vi "Read files V CH1(Recorder).vi"(10 "Path":path, 11 "Number":dbl) -> (3 "Voltage":dbl format="%_5g")   [LabVIEW 2020, in "GPP.lvlib"]
uses:
  GPP.lvlib
panel:
  out "String":string
  out "String 2":string
  out "String 3":string
  out "Array":u8[](array[numeric])
  out "Numeric":u16
  out "V1 2":string
  out "V1":string
  out "LAST1":string
  out "SET":string
  out "ALL":string
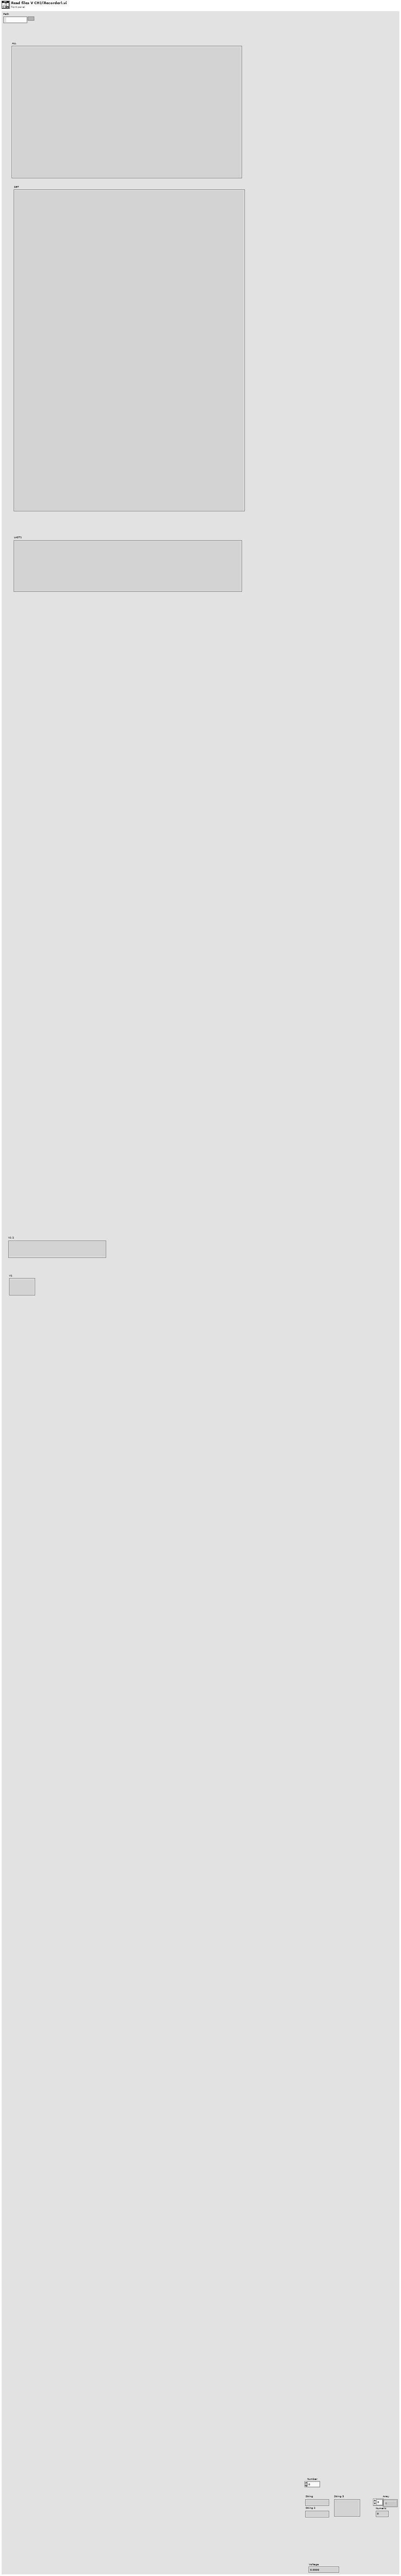
[diagram p1: front panel]
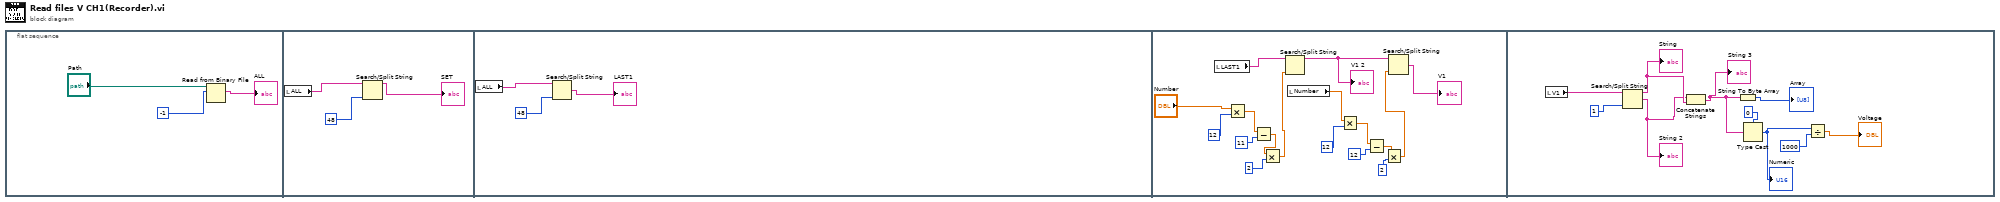
[diagram p0: block diagram]
diagram:
  n1 = flat-sequence {
    frame #0 {
      n2 = Read from Binary File(10:-1, 11:"Path") -> (2:→"ALL":string)  [unwired: 4 in, 3 out]
    }
    frame #1 {
      n3 = local read "ALL"() -> (w4:string)
      n4 = Search/Split String(string=w4, offset (0)=48) -> (substring before match=→"SET":string)  [unwired: 1 in, 2 out]
    }
    frame #2 {
      n5 = local read "ALL"() -> (w7:string)
      n6 = Search/Split String(string=w7, offset (0)=48) -> (match + rest of string=→"LAST1":string)  [unwired: 1 in, 2 out]
    }
    frame #3 {
      n7 = local read "LAST1"() -> (w23:string)
      n8 = Multiply(x="Number", y=12) -> (x*y=w22:dbl)
      n9 = Subtract(x=w22, y=11) -> (x-y=w15:dbl)
      n10 = Multiply(x=w15, y=2) -> (x*y=w13:dbl)
      n11 = Search/Split String(string=w23, offset (0)=w13) -> (substring before match=w16:string)  [unwired: 1 in, 2 out]
      "V1 2" <- w16
      n12 = local read "Number"() -> (w17:dbl)
      n13 = Multiply(x=w17, y=12) -> (x*y=w19:dbl)
      n14 = Subtract(x=w19, y=12) -> (x-y=w12:dbl)
      n15 = Multiply(x=w12, y=2) -> (x*y=w10:dbl)
      n16 = Search/Split String(string=w16, offset (0)=w10) -> (match + rest of string=→"V1":string)  [unwired: 1 in, 2 out]
    }
    frame #4 {
      n17 = local read "V1"() -> (w36:string)
      n18 = Search/Split String(string=w36, offset (0)=1) -> (substring before match=w34:string, match + rest of string=w33:string)  [unwired: 1 in, 1 out]
      "String" <- w34
      "String 2" <- w33
      n19 = Concatenate Strings(w33, w34) -> (w31:string)
      "String 3" <- w31
      n20 = String To Byte Array(string=w31) -> (unsigned byte array=→"Array":u8[])
      n21 = Type Cast(type=u16 0, x=w31) -> (*(type *) &x=w29:u16)
      "Numeric" <- w29
      n22 = Divide(x=w29, y=1000) -> (x/y=→"Voltage":dbl)
    }
  }
